vi "Backup Nim test database from last save.vi"(8 "error in (no error)":errorcluster) -> (0 "error out":errorcluster, 2 "New test recs":i32, 3 "Curr test rec cnt":i32)   [LabVIEW 2013]
uses:
  <vilib>/Utility/file.llb/Read From Spreadsheet File (string).vi
  <vilib>/Utility/file.llb/Write To Spreadsheet File (string).vi
panel:
  out "Recs":i32
  out "Used file path":path
  out "Last line":string[](array[string])
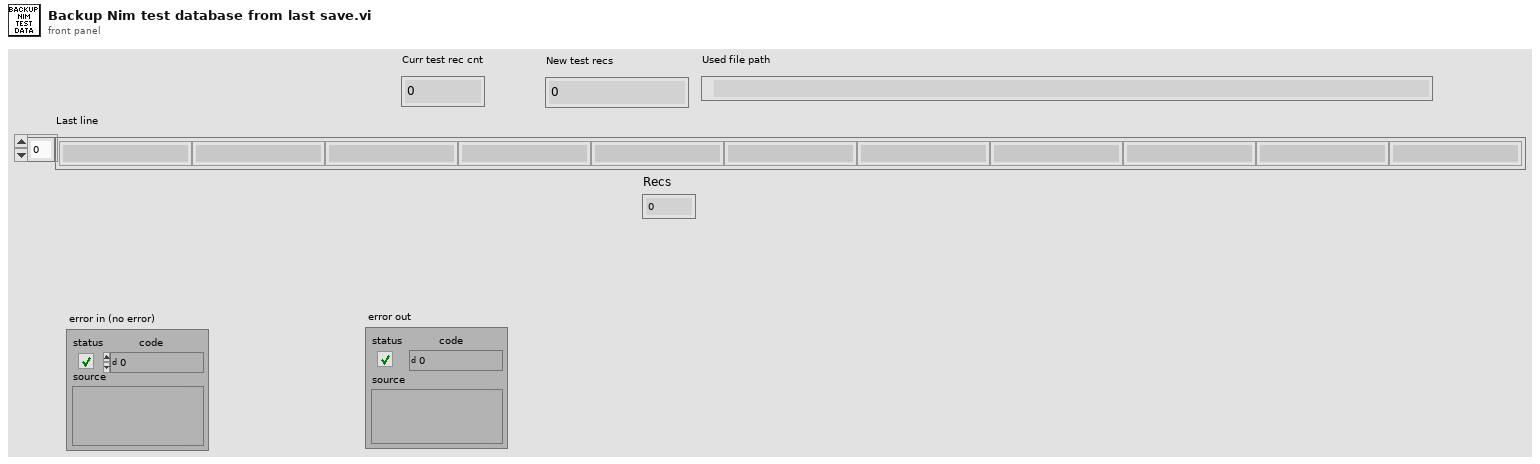
[diagram p1: front panel]
types:
  T1 = enum16{"Query", "Insert", "Select", "Dump Recs", "Get Rec Count", "Get Col Names", "Insert all fields", "Find", "Get last test result", "Get work order qty", "Set work order qty", "Save test report", "Get test report", "Execute query no data", "Select count", "Query and return row 0 col 0"}
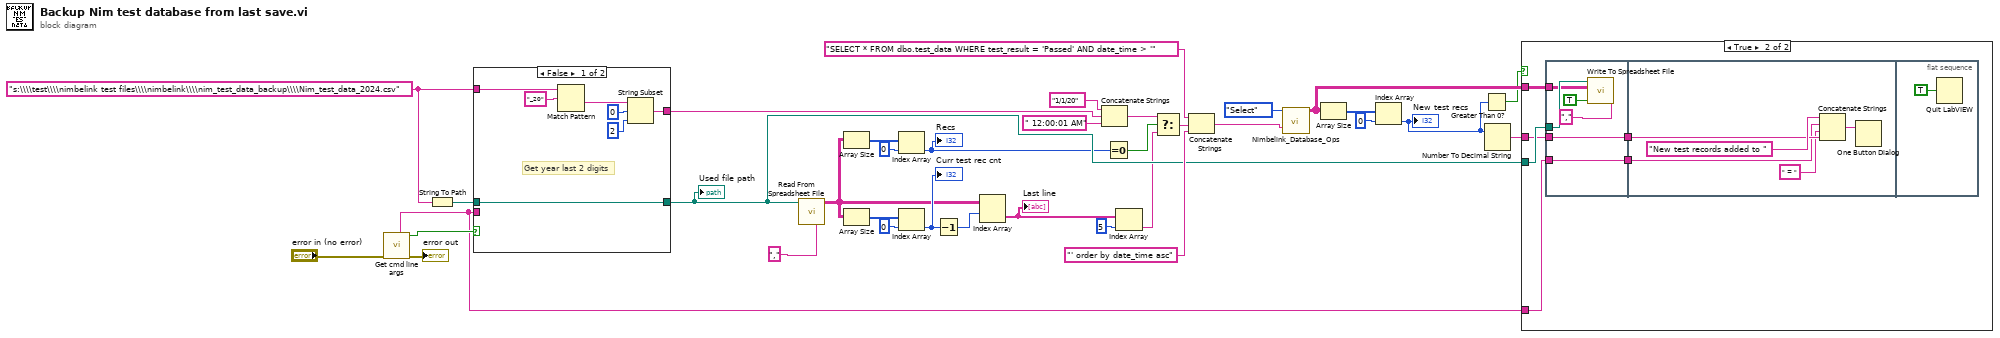
[diagram p0: block diagram]
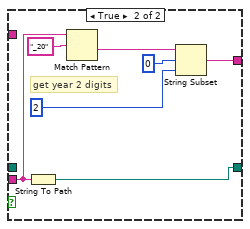
[diagram p2: hidden frame]
diagram:
  w7 = "s:\\\\test\\\\nimbelink test files\\\\nimbelink\\\\nim_test_data_backup\\\\Nim_test_data_2024.csv"
  n1 = call "Get cmd line args.vi"("error in (no error)"="error in (no error)") -> ("error out"=→"error out":errorcluster, "Got cmd line args?"=w16:bool, "arg1"=w14:string)  [unwired: 3 in, 5 out]
  n2 = String To Path(string=w7) -> (path=w13:path)
  n3 = case shown="False" w16 {
    tunnel: w14 -> [_ w48]
    tunnel: [w42 w49] -> w15
    tunnel: w13 -> [w42 _]
    tunnel: [w36 w43] -> w5
    tunnel: w7 -> [w37 _]
    frame False {
      # "Get year last 2 digits"
      n4 = Match Pattern(string=w37, regular expression="_20") -> (after substring=w38:string)  [unwired: 1 in, 3 out]
      n5 = String Subset(string=w38, offset (0)=0, length (rest)=2 ("length (rest)")) -> (substring=w36:string)
    }
    frame True {
      # "get year 2 digits"
      n6 = String To Path(string=w48) -> (path=w49:path)
      n7 = Match Pattern(string=w48, regular expression="_20") -> (after substring=w44:string)  [unwired: 1 in, 3 out]
      n8 = String Subset(string=w44, offset (0)=0, length (rest)=2 ("length (rest)")) -> (substring=w43:string)
    }
  }
  "Used file path" <- w15
  n9 = call-poly <vilib>:"Read From Spreadsheet File.vi"("delimiter (\\t)"="," ("delimiter (\\t)"), "file path (dialog if empty)"=w15) -> ("all rows"=w12:string[][])  [unwired: 5 in, 4 out]
  n10 = Array Size(array=w12) -> (size(s)=w11:i32[])
  n11 = Array Size(array=w12) -> (size(s)=w34:i32[])
  n12 = Index Array(array=w11, index=0) -> (element=w8:i32)
  "Recs" <- w8
  n13 = Index Array(array=w34, index=0) -> (element=w32:i32)
  "Curr test rec cnt" <- w32
  n14 = Decrement(x=w32) -> (x-1=w31:i32)
  n15 = Index Array(array=w12, index (row)=w31) -> (element=w29:string[])  [unwired: 1 in]
  "Last line" <- w29
  n16 = Concatenate Strings("1/1/20", w5, " 12:00:01 AM" ("string")) -> (w3:string)
  n17 = Equal To 0?(x=w8) -> (x = 0?=w9:bool)
  n18 = Index Array(array=w29, index=5) -> (element=w2:string)
  n19 = Select(t=w3, s=w9, f=w2) -> (s? t:f=w1:string)
  n20 = Concatenate Strings("SELECT * FROM dbo.test_data WHERE test_result = 'Passed' AND date_time > '" ("SQL Query"), w1, "' order by date_time asc" ("string")) -> (w25:string)
  n21 = call "Nimbelink_Database_Ops.vi"("Operation"=T1."Select", "SQL Query"=w25) -> ("RecordSet"=w24:string[][])  [unwired: 10 in, 7 out]
  n22 = Array Size(array=w24) -> (size(s)=w23:i32[])
  n23 = Index Array(array=w23, index=0) -> (element=w20:i32)
  "New test recs" <- w20
  n24 = Greater Than 0?(x=w20) -> (x > 0?=w21:bool)
  n25 = Number To Decimal String(number=w20) -> (decimal integer string=w19:string)  [unwired: 1 in]
  n26 = case shown="True" w21 {
    tunnel: w15 -> [_ w55]
    tunnel: w24 -> [_ w54]
    tunnel: w19 -> [_ w52]
    tunnel: w14 -> [_ w50]
    frame False {
    }
    frame True {
      n27 = flat-sequence {
        tunnel: w55 -> [w59]
        tunnel: w54 -> [w58]
        tunnel: [w57] -> w53
        tunnel: w52 -> [w57]
        tunnel: [w56] -> w51
        tunnel: w50 -> [w56]
        tunnel: w53 -> [w64]
        tunnel: w51 -> [w63]
        frame #0 {
          n28 = call-poly <vilib>:"Write To Spreadsheet File.vi"("delimiter (\\t)"="," ("delimiter (\\t)"), "append to file? (new file:F)"=TRUE, "2D data"=w58, "file path (dialog if empty)"=w59) -> ()  [unwired: 4 in, 1 out]
        }
        frame #1 {
          n29 = Concatenate Strings("New test records added to " ("string"), w63, " = " ("string"), w64) -> (w66:string)
          n30 = One Button Dialog(message=w66) -> ()  [unwired: 1 in, 1 out]
        }
        frame #2 {
          n31 = Quit LabVIEW(quit? (T)=TRUE) -> ()
        }
      }
    }
  }
